vi "Configure Voltage1.vi"(7 "Voltage Integration Time (10: 10)":dbl(ring)=10.0 items=["0.02"=0.02, "0.2"=0.2, "1"=1.0, "10"=10.0, "100"=100.0], 8 "error in (no error)":errorcluster, 9 "Auto Impedance (F: Disable)":bool, 10 "Voltage Bandwidth (20: 20 Hz)":i32(ring)=20 items=["3"=3, "20"=20, "200"=200], 11 "VISA resource name":refnum<visa-resource-name>) -> (0 "error out":errorcluster, 3 "VISA resource name out":refnum<visa-resource-name>)   [LabVIEW 2015, in "Agilent 3446X Series1.lvlib"]
doc: "Configures the settings for voltage measurements."
uses:
  Agilent 3446X Series1.lvlib
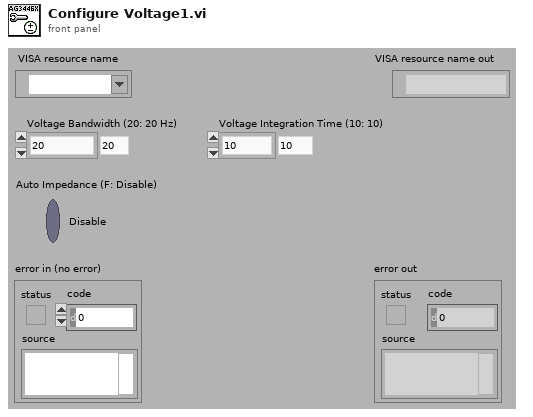
[diagram p1: front panel]
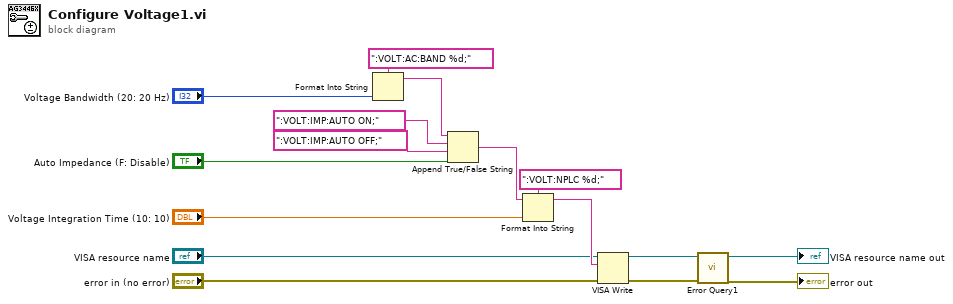
[diagram p0: block diagram]
diagram:
  n1 = Format Into String(format string=":VOLT:AC:BAND %d;", "Voltage Bandwidth (20: 20 Hz)") -> (resulting string=w14:string)  [unwired: 2 in, 1 out]
  n2 = Append True/False String(1:"Auto Impedance (F: Disable)", 2:":VOLT:IMP:AUTO OFF;", 3:":VOLT:IMP:AUTO ON;", 4:w14) -> (0:w10:string)
  n3 = Format Into String(format string=":VOLT:NPLC %d;", initial string=w10, "Voltage Integration Time (10: 10)") -> (resulting string=w7:string)  [unwired: 1 in, 1 out]
  n4 = VISA Write(VISA resource name="VISA resource name", write buffer=w7, error in (no error)="error in (no error)") -> (VISA resource name out=w4:refnum<visa-resource-name>, error out=w3:errorcluster)  [unwired: 1 out]
  n5 = call "Error Query1.vi"("error in (no error)"=w3, "VISA resource name"=w4) -> ("error out"=→"error out":errorcluster, "VISA resource name out"=→"VISA resource name out":refnum<visa-resource-name>)  [unwired: 8 out]
